vi "Build Info.vi"(8 "error in (no error)":errorcluster, 11 "Simple Build GUI in":refnum<class "Simple Build GUI.lvclass">) -> (0 "error out":errorcluster, 1 "Builds":T1[](array[typedef]), 2 "Project":string, 3 "Simple Build GUI out":refnum<class "Simple Build GUI.lvclass">)   [LabVIEW 2020, in "Builder Tools.lvlib" / "Simple Build GUI.lvclass"]
uses:
  Simple Build GUI.lvclass
  Build Info.ctl
  Simple Build GUI.lvclass/Simple Build GUI.ctl
  Builder/Builder.lvclass
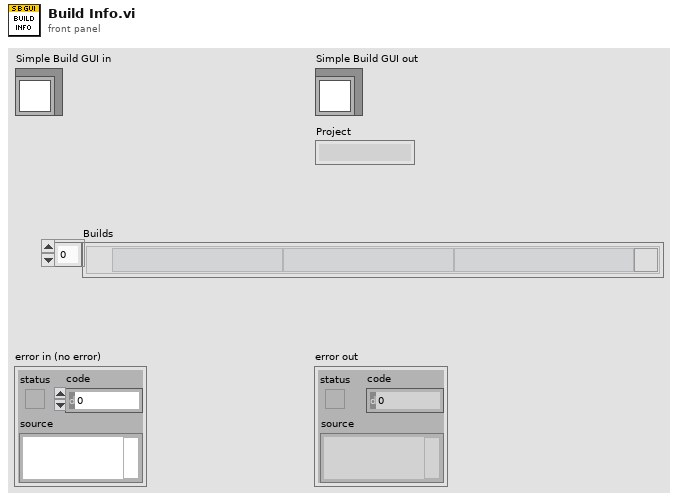
[diagram p1: front panel]
types:
  T1 = typedef "Builder Tools.lvlib/Simple Build GUI.lvclass/Build Info.ctl" = cluster{"Picture":picture, "Project":string, "Target":string, "Build Spec":string, "Build":bool}
  T2 = typedef "Builder Tools.lvlib/Build Info.ctl" = cluster{"Project Path":path, "Target":string, "Build Spec":string}
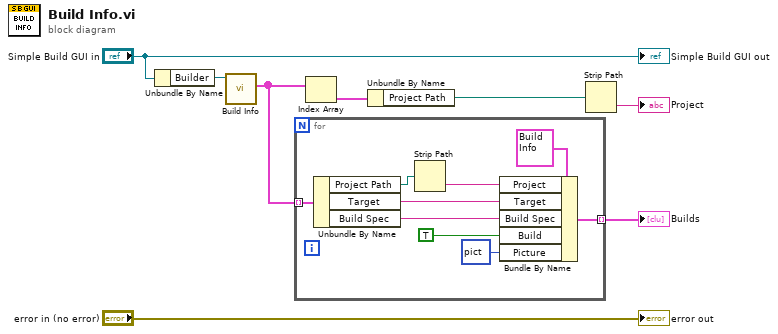
[diagram p0: block diagram]
diagram:
  n1 = Unbundle By Name("Simple Build GUI in") -> ("Builder"=w6:refnum<class "Builder.lvclass">)
  n2 = call "Build Info.vi"("Builder in"=w6) -> ("Build Info"=w2:T2[])  [unwired: 9 in, 1 out]
  n3 = for {
    tunnel: w2 -> [w17] mode=indexing
    tunnel: [w13] -> w1 mode=indexing
    n4 = Unbundle By Name(w17) -> ("Project Path"=w12:path, "Target"=w16:string, "Build Spec"=w15:string)
    n5 = Strip Path(path=w12) -> (name=w11:string)  [unwired: 1 out]
    n6 = Bundle By Name(cluster=T1 {"Picture"=bytes[0], "Project"="", "Target"="", "Build Spec"="", "Build"=FALSE} ("Build Info"), "Project"=w11, "Target"=w16, "Build Spec"=w15, "Build"=TRUE, "Picture"=picture data[5B]) -> (w13:T1)
  }
  "Builds" <- w1
  n7 = Index Array(array=w2) -> (element=w5:T2)  [unwired: 1 in]
  n8 = Unbundle By Name(w5) -> ("Project Path"=w4:path)
  n9 = Strip Path(path=w4) -> (name=→"Project":string)  [unwired: 1 out]
  "error out" <- "error in (no error)"
  "Simple Build GUI out" <- "Simple Build GUI in"
